vi "reading to mag reading.vi"(4 "magnetometer y locations":dbl[](array[numeric])=[0.0, 38.971, -38.971, 0.0], 6 "magnetometer x locations":dbl[](array[numeric])=[0.0, -22.5, -22.5, 45.0], 9 "reading":T2) -> (1 "mag reading":T1)   [LabVIEW 2017]
uses:
  typedefs/reading.ctl
  typedefs/readingType.ctl
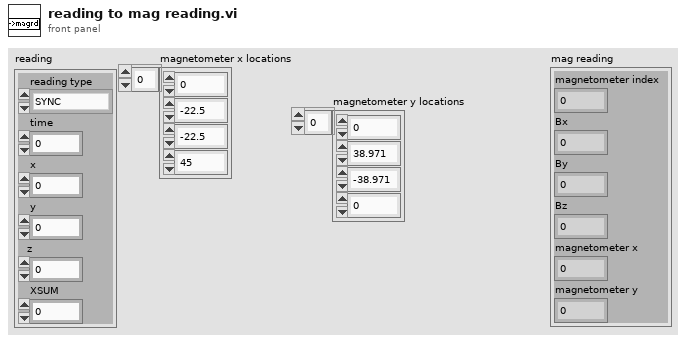
[diagram p1: front panel]
types:
  T1 = cluster{"magnetometer index":dbl, "Bx":dbl, "By":dbl, "Bz":dbl, "magnetometer x":dbl, "magnetometer y":dbl}
  T2 = typedef "reading.ctl" = cluster{"reading type":T3, "time":fxp<+,48,48>, "x":sgl, "y":sgl, "z":sgl, "XSUM":u8}
  T3 = typedef "readingType.ctl" = enum8{"SYNC", "DETVAL", "COILI", "MAGVEC", "ACCVEC", "CROSSING", "MAGVEC0", "MAGVEC1", "MAGVEC2", "MAGVEC3", "MAGVEC4", "MAGVEC5", "MAGVEC6", "MAGVEC7"}
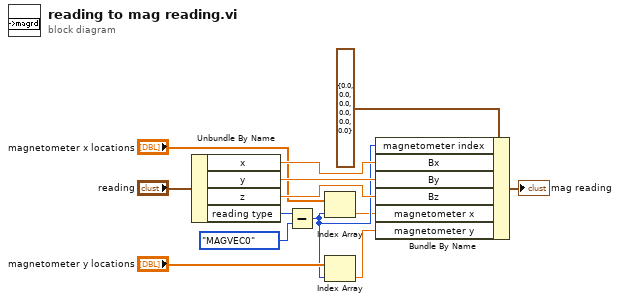
[diagram p0: block diagram]
diagram:
  n1 = Unbundle By Name("reading") -> ("x"=w11:sgl, "y"=w10:sgl, "z"=w9:sgl, "reading type"=w8:T3)
  n2 = Subtract(x=w8, y=readingType."MAGVEC0") -> (x-y=w3:u8)
  n3 = Index Array(array="magnetometer x locations", index=w3) -> (element=w2:dbl)
  n4 = Index Array(array="magnetometer y locations", index=w3) -> (element=w5:dbl)
  n5 = Bundle By Name(cluster=T1 {"magnetometer index"=0.0, "Bx"=0.0, "By"=0.0, "Bz"=0.0, "magnetometer x"=0.0, "magnetometer y"=0.0} ("mag readings"), "magnetometer index"=w3, "Bx"=w11, "By"=w10, "Bz"=w9, "magnetometer x"=w2, "magnetometer y"=w5) -> (→"mag reading":T1)
